vi "templates PLOTS data keys.vi"(9 "Template Keys":T1, 10 "HTM Keys":T1) -> (2 "HTM Keys":T1)   [LabVIEW 2011]
uses:
  ITK EXT/utils/keyedarr.llb/Keyed Array.ctl
  ITK EXT/utils/strutil.llb/Case Matching.ctl
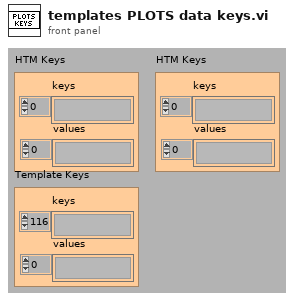
[diagram p1: front panel]
types:
  T1 = typedef "Keyed Array.ctl" = cluster{"keys":string[], "values":string[]}
  T2 = typedef "Case Matching.ctl" = enum16{"a != A", "a == A", "system"}
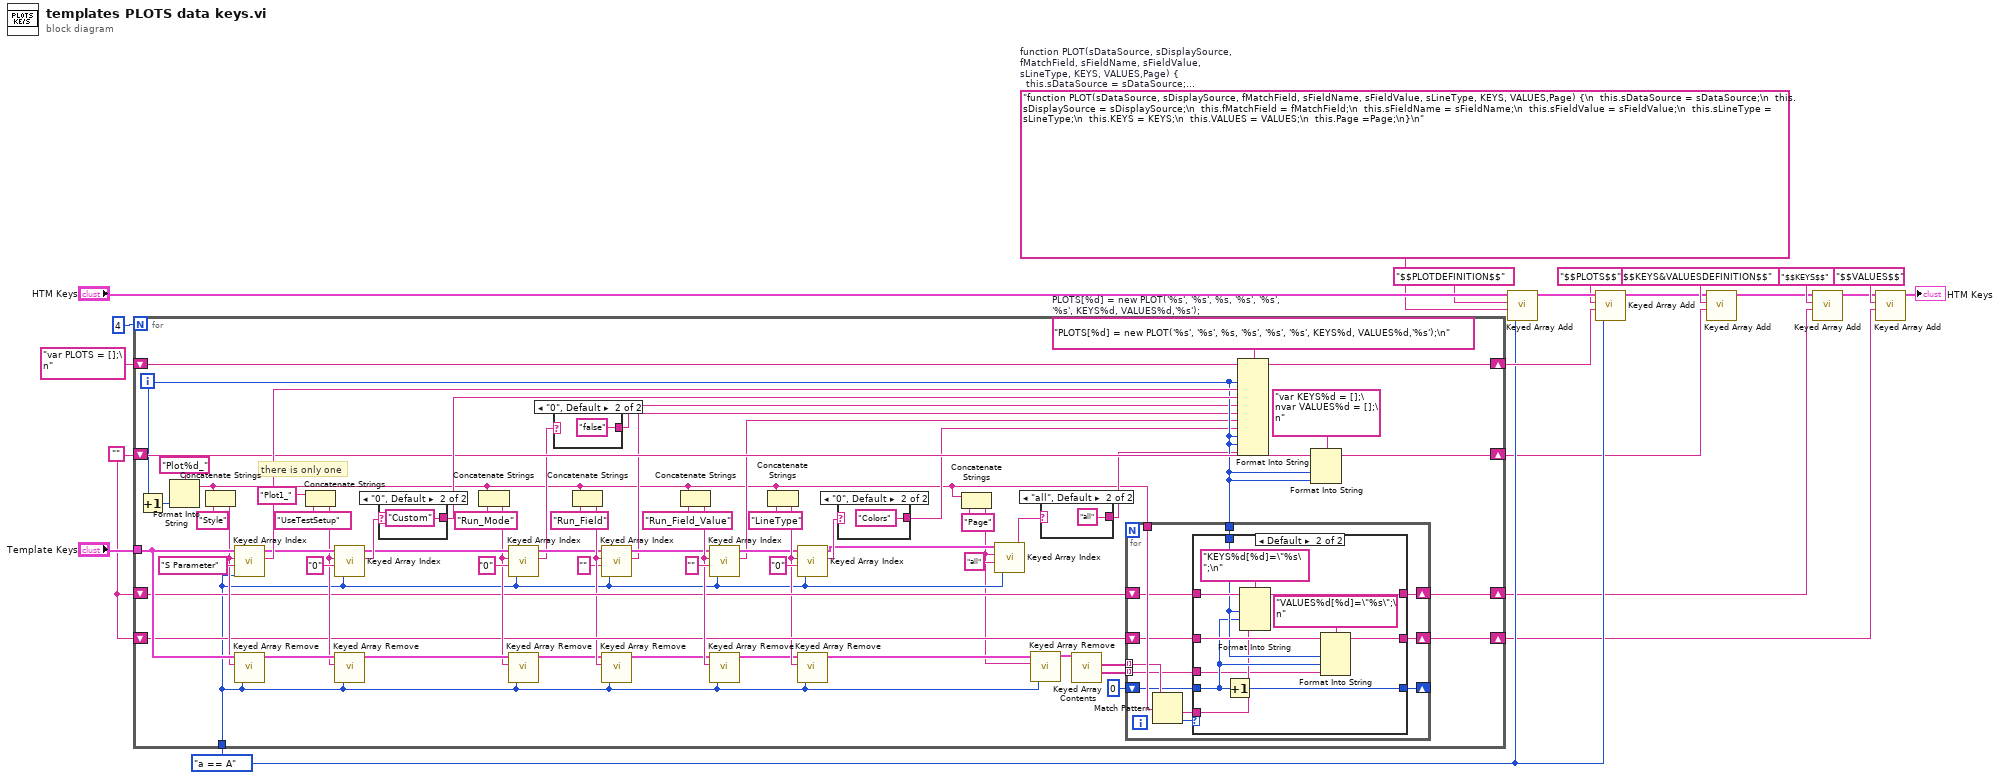
[diagram p0: block diagram]
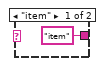
[diagram p2: hidden frame]
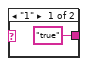
[diagram p3: hidden frame]
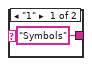
[diagram p4: hidden frame]
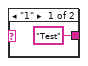
[diagram p6: hidden frame]
diagram:
  w11 = ""
  w12 = Case_Matching."a == A" ("case matching (sensitive)")
  w17 = "function PLOT(sDataSource, sDisplaySource, fMatchField, sFieldName, sFieldValue, sLineType, KEYS, VALUES,Page) {\n  this.sDataSource = sDataSource;\n  this.sDisplaySource = sDisplaySource;\n  this.fMatchField = fMatchField;\n  this.sFieldName = sFieldName;\n  this.sFieldValue = sFieldValue;\n  this.sLineType = sLineType;\n  this.KEYS = KEYS;\n  this.VALUES = VALUES;\n  this.Page =Page;\n}\n"  # function PLOT(sDataSource, sDisplaySource, fMatchField, sFieldName, sFieldValue, sLineType, KEYS, VALUES,Page) {   this.sDataSource = sDataSource;   this.sDisplaySource = sDisplaySource;   this.fMatchField = fMatchField;   this.sFieldName = sFieldName;   this.sFieldValue = sFieldValue;   this.sLineType = sLineType;   this.KEYS = KEYS;   this.VALUES = VALUES;   this.Page =Page; }
  n1 = for {
    N: 4 -> [_]
    shift-right: [w84] -> w14
    shift-left: "var PLOTS = [];\n" ("format string") -> [w85]
    tunnel: "Template Keys" -> [w68]
    tunnel: w12 -> [w26]
    shift-right: [w59] -> w3
    shift-left: w11 -> [w58]
    shift-right: [w56] -> w1
    shift-left: w11 -> [w55]
    shift-right: [w57] -> w2
    shift-left: w11 -> [w54]
    i -> [w36]
    w86 = "PLOTS[%d] = new PLOT('%s', '%s', %s, '%s', '%s', '%s', KEYS%d, VALUES%d,'%s');\n"  # PLOTS[%d] = new PLOT('%s', '%s', %s, '%s', '%s', '%s', KEYS%d, VALUES%d,'%s');
    # "there is only one"
    n2 = Increment(x=w36) -> (x+1=w83:i32)
    n3 = Format Into String(format string="Plot%d_", w83) -> (resulting string=w23:string)  [unwired: 2 in, 1 out]
    n4 = Concatenate Strings(w23, "Style" ("format string")) -> (w65:string)
    n5 = call "Keyed Array Index.vi"("case matching (sensitive)"=w26, "default value"="S Parameter", "key"=w65, "array in"=w68) -> ("value"=w79:string, "duplicate array"=w78:T1)  [unwired: 2 out]
    n6 = call "Keyed Array Remove.vi"("case matching (sensitive)"=w26, "key"=w65, "array in"=w68) -> ("array out"=w67:T1)  [unwired: 4 out]
    n7 = Concatenate Strings("Plot1_" ("format string"), "UseTestSetup" ("format string")) -> (w64:string)
    n8 = call "Keyed Array Index.vi"("case matching (sensitive)"=w26, "default value"="0", "key"=w64, "array in"=w78) -> ("value"=w75:string, "duplicate array"=w72:T1)  [unwired: 2 out]
    n9 = call "Keyed Array Remove.vi"("case matching (sensitive)"=w26, "key"=w64, "array in"=w67) -> ("array out"=w66:T1)  [unwired: 4 out]
    n10 = case shown="\"0\", Default" w75 {
      tunnel: ["Test" ("default value") "Custom" ("default value")] -> w74
      frame "1" {
      }
      frame "0", Default {
      }
    }
    n11 = Concatenate Strings(w23, "Run_Mode" ("format string")) -> (w63:string)
    n12 = call "Keyed Array Index.vi"("case matching (sensitive)"=w26, "default value"="0" ("format string"), "key"=w63, "array in"=w72) -> ("value"=w37:string, "duplicate array"=w38:T1)  [unwired: 2 out]
    n13 = call "Keyed Array Remove.vi"("case matching (sensitive)"=w26, "key"=w63, "array in"=w66) -> ("array out"=w41:T1)  [unwired: 4 out]
    n14 = case shown="\"0\", Default" w37 {
      tunnel: ["true" ("default value") "false" ("default value")] -> w35
      frame "1" {
      }
      frame "0", Default {
      }
    }
    n15 = Concatenate Strings(w23, "Run_Field" ("format string")) -> (w44:string)
    n16 = call "Keyed Array Index.vi"("case matching (sensitive)"=w26, "default value"="" ("format string"), "key"=w44, "array in"=w38) -> ("value"=w34:string, "duplicate array"=w39:T1)  [unwired: 2 out]
    n17 = call "Keyed Array Remove.vi"("case matching (sensitive)"=w26, "key"=w44, "array in"=w41) -> ("array out"=w40:T1)  [unwired: 4 out]
    n18 = Concatenate Strings(w23, "Run_Field_Value" ("format string")) -> (w62:string)
    n19 = call "Keyed Array Index.vi"("case matching (sensitive)"=w26, "default value"="" ("format string"), "key"=w62, "array in"=w39) -> ("value"=w33:string, "duplicate array"=w48:T1)  [unwired: 2 out]
    n20 = call "Keyed Array Remove.vi"("case matching (sensitive)"=w26, "key"=w62, "array in"=w40) -> ("array out"=w47:T1)  [unwired: 4 out]
    n21 = Concatenate Strings(w23, "LineType" ("format string")) -> (w49:string)
    n22 = call "Keyed Array Index.vi"("case matching (sensitive)"=w26, "default value"="0" ("format string"), "key"=w49, "array in"=w48) -> ("value"=w46:string, "duplicate array"=w29:T1)  [unwired: 2 out]
    n23 = call "Keyed Array Remove.vi"("case matching (sensitive)"=w26, "key"=w49, "array in"=w47) -> ("array out"=w27:T1)  [unwired: 4 out]
    n24 = case shown="\"0\", Default" w46 {
      tunnel: ["Symbols" ("default value") "Colors" ("default value")] -> w32
      frame "1" {
      }
      frame "0", Default {
      }
    }
    n25 = Concatenate Strings(w23, "Page" ("format string")) -> (w22:string)
    n26 = call "Keyed Array Index.vi"("case matching (sensitive)"=w26, "default value"="all" ("format string"), "key"=w22, "array in"=w29) -> ("value"=w28:string)  [unwired: 3 out]
    n27 = call "Keyed Array Remove.vi"("case matching (sensitive)"=w26, "key"=w22, "array in"=w27) -> ("array out"=w25:T1)  [unwired: 4 out]
    n28 = case shown="\"all\", Default" w28 {
      tunnel: ["item" ("default value") "all" ("default value")] -> w31
      frame "item" {
      }
      frame "all", Default {
      }
    }
    n29 = call "Keyed Array Contents.vi"("array in"=w25) -> ("values"=w52:string[], "keys"=w53:string[])  [unwired: 5 out]
    n30 = for {
      tunnel: w53 -> [w102] mode=indexing
      tunnel: w23 -> [w104]
      shift-right: [w100] -> w57
      shift-left: w54 -> [w101]
      tunnel: w52 -> [w99] mode=indexing
      shift-right: [w97] -> w56
      shift-left: w55 -> [w98]
      shift-right: [w95] -> _
      shift-left: 0 -> [w96]
      tunnel: w36 -> [w94]
      n31 = Match Pattern(string=w102, regular expression=w104) -> (after substring=w93:string, offset past match=w103:i32)  [unwired: 3 out]
      n32 = case shown="Default" w103 {
        tunnel: w101 -> [w107 w118]
        tunnel: [w107 w117] -> w100
        tunnel: w99 -> [_ w108]
        tunnel: w98 -> [w106 w116]
        tunnel: [w106 w115] -> w97
        tunnel: w96 -> [w105 w110]
        tunnel: [w105 w112] -> w95
        tunnel: w94 -> [_ w111]
        tunnel: w93 -> [_ w109]
        frame -1 {
        }
        frame Default {
          n33 = Increment(x=w110) -> (x+1=w112:i32)
          n34 = Format Into String(format string="KEYS%d[%d]=\"%s\";\n", initial string=w118, w111, w110, w109) -> (resulting string=w117:string)  [unwired: 1 in, 1 out]
          n35 = Format Into String(format string="VALUES%d[%d]=\"%s\";\n", initial string=w116, w111, w110, w108) -> (resulting string=w115:string)  [unwired: 1 in, 1 out]
        }
      }
    }
    n36 = Format Into String(format string=w86, initial string=w85, w36, w79, w74, w35, w34, w33, w32, w36, w36, w31) -> (resulting string=w84:string)  [unwired: 1 in, 1 out]
    n37 = Format Into String(format string="var KEYS%d = [];\nvar VALUES%d = [];\n", initial string=w58, w36, w36) -> (resulting string=w59:string)  [unwired: 1 in, 1 out]
  }
  n38 = call "Keyed Array Add.vi"("case matching (sensitive)"=w12, "value"=w17, "key"="$$PLOTDEFINITION$$", "array in"="HTM Keys") -> ("array out"=w16:T1)  [unwired: 3 out]
  n39 = call "Keyed Array Add.vi"("case matching (sensitive)"=w12, "value"=w14, "key"="$$PLOTS$$", "array in"=w16) -> ("array out"=w4:T1)  [unwired: 3 out]
  n40 = call "Keyed Array Add.vi"("value"=w3, "key"="$$KEYS&VALUESDEFINITION$$", "array in"=w4) -> ("array out"=w7:T1)  [unwired: 1 in, 3 out]
  n41 = call "Keyed Array Add.vi"("value"=w2, "key"="$$KEYS$$", "array in"=w7) -> ("array out"=w6:T1)  [unwired: 1 in, 3 out]
  n42 = call "Keyed Array Add.vi"("value"=w1, "key"="$$VALUES$$", "array in"=w6) -> ("array out"=→"HTM Keys":T1)  [unwired: 1 in, 3 out]
